vi "Set_Parameter_Instrument (Json).vi"(8 "error in (no error)":errorcluster caption="entrée d'erreur (pas d'erreur)", 10 "Parameter (Json)":string, 11 "Enable_DIO en entrée":refnum<class "Start_Continuous_Ana.lvclass">) -> (0 "error out":errorcluster caption="sortie d'erreur", 3 "Enable_DIO en sortie":refnum<class "Start_Continuous_Ana.lvclass">)   [LabVIEW 2020, in "Library Test.lvlib" / "Start_Continuous_Ana.lvclass"]
uses:
  Start_Continuous_Ana.lvclass
  C:/Users/ngarcin/OneDrive - Altyor/Standard TB/Class/Test/Test (Default)/Test (Default).lvclass
  Ana/Class Ana (Default)/Class Ana (Default).lvclass
  JSON API/JSON Value/Set from JSON string.vi
  JSON API/Variant JSON/Variant to JSON.vi
  JSON API/JSON Value/Get Item by name array.vi
  Test_Wtih_Instr/Test_With_Inst.lvclass
  Instrument/Instrument (Default)/Class Instrument (Default).lvclass
  JSON API/JSON Value/JSON Value.lvclass
  Start_Continuous_Ana.lvclass/Start_Continuous_Ana.ctl
  JSON API/Variant JSON/Variant JSON.lvlib
  JSON API/Get Polymorphic/JSON GetSet.lvlib
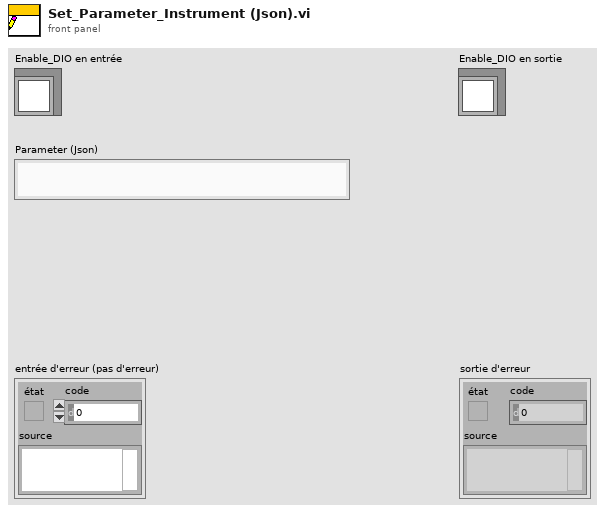
[diagram p1: front panel]
types:
  T1 = cluster{"Device_Com_Port":string, "Rate":u16, "Nb Sample":u16, "Voltage Max":dbl, "Voltage Min":dbl, "Input terminal Configuration":string, "Channel":u8[], "Continuous":bool, "Nb Data_To_Read":i16, "Class Ana":refnum<class "Class Ana (Default).lvclass">}
  T2 = cluster{"Rate":u16, "Nb Sample":u16, "Voltage Max":dbl, "Voltage Min":dbl, "Input terminal Configuration":string, "Channel":u8[], "Nb Data_To_Read":i16}
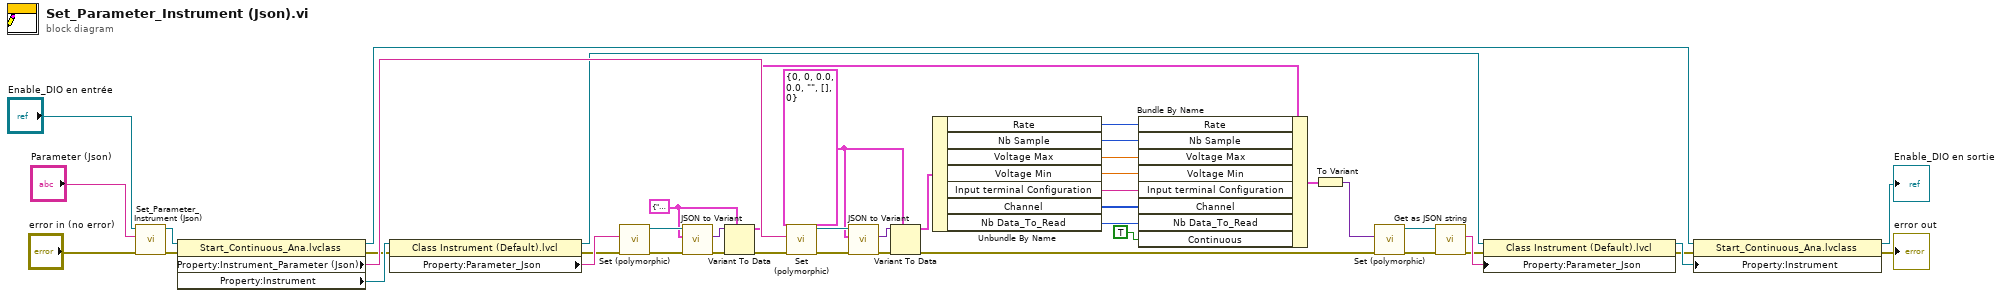
[diagram p0: block diagram]
diagram:
  w6 = T1 {"Device_Com_Port"="", "Rate"=0, "Nb Sample"=0, "Voltage Max"=0.0, "Voltage Min"=0.0, "Input terminal Configuration"="", "Channel"=[], "Continuous"=FALSE, "Nb Data_To_Read"=0, "Class Ana"=refnum} ("Parameter")
  w8 = T2 {"Rate"=0, "Nb Sample"=0, "Voltage Max"=0.0, "Voltage Min"=0.0, "Input terminal Configuration"="", "Channel"=[], "Nb Data_To_Read"=0} ("Parameter")
  n1 = call-parent "Set_Parameter_Instrument (Json).vi"("error in (no error)"="error in (no error)", "Parameter (Json)"="Parameter (Json)", "Test (Default) en entrée"="Enable_DIO en entrée") -> ("error out"=w19:errorcluster, "Test (Default) en sortie"=w27:refnum<class "Start_Continuous_Ana.lvclass">)  [unwired: 7 in]
  n2 = property class="Start_Continuous_Ana.lvclass"(reference=w27, error in=w19) -> (reference out=w23:refnum<class "Start_Continuous_Ana.lvclass">, error out=w18:errorcluster, "Property:Instrument_Parameter (Json)"=w25:string, "Property:Instrument"=w26:refnum<class "Class Instrument (Default).lvclass">)
  n3 = property class="Class Instrument (Default).lvcl"(reference=w26, error in=w18) -> (reference out=w22:refnum<class "Class Instrument (Default).lvclass">, error out=w31:errorcluster, "Property:Parameter_Json"=w33:string)
  n4 = call-poly "Set (polymorphic).vi"("error in (no error)"=w31, "JSON stream"=w33) -> ("error out"=w35:errorcluster, "JSON Value out"=w37:refnum<class "JSON Value.lvclass">)  [unwired: 7 in, 1 out]
  n5 = call "JSON to Variant.vi"("error in (no error)"=w35, "Variant (Data Type)"=w6, "JSON Value"=w37) -> ("error out"=w36:errorcluster, "Variant out"=w34:variant)  [unwired: 7 in]
  n6 = Variant To Data(error in=w36, type=w6, Variant=w34) -> (data=w1:T1, error out=w32:errorcluster)
  n7 = call-poly "Set (polymorphic).vi"("error in (no error)"=w32, "JSON stream"=w25) -> ("error out"=w40:errorcluster, "JSON Value out"=w38:refnum<class "JSON Value.lvclass">)  [unwired: 7 in, 1 out]
  n8 = call "JSON to Variant.vi"("error in (no error)"=w40, "Variant (Data Type)"=w8, "JSON Value"=w38) -> ("error out"=w39:errorcluster, "Variant out"=w41:variant)  [unwired: 7 in]
  n9 = Variant To Data(error in=w39, type=w8, Variant=w41) -> (data=w7:T2, error out=w4:errorcluster)
  n10 = Unbundle By Name(w7) -> ("Rate"=w16:u16, "Nb Sample"=w15:u16, "Voltage Max"=w14:dbl, "Voltage Min"=w13:dbl, "Input terminal Configuration"=w12:string, "Channel"=w11:u8[], "Nb Data_To_Read"=w10:i16)
  n11 = Bundle By Name(cluster=w1, "Rate"=w16, "Nb Sample"=w15, "Voltage Max"=w14, "Voltage Min"=w13, "Input terminal Configuration"=w12, "Channel"=w11, "Nb Data_To_Read"=w10, "Continuous"=TRUE) -> (w5:T1)
  n12 = To Variant(anything=w5) -> (Variant=w29:variant)
  n13 = call-poly "Set (polymorphic).vi"("error in (no error)"=w4, "Variant"=w29) -> ("error out"=w3:errorcluster, "JSON Value out"=w30:refnum<class "JSON Value.lvclass">)  [unwired: 8 in]
  n14 = call "Get as JSON string.vi"("error in (no error)"=w3, "JSON Value in"=w30) -> ("error out"=w2:errorcluster, "<JSON>"=w28:string)  [unwired: 8 in]
  n15 = property class="Class Instrument (Default).lvcl"(reference=w22, error in=w2, "Property:Parameter_Json"=w28) -> (reference out=w24:refnum<class "Class Instrument (Default).lvclass">, error out=w17:errorcluster)
  n16 = property class="Start_Continuous_Ana.lvclass"(reference=w23, error in=w17, "Property:Instrument"=w24) -> (reference out=→"Enable_DIO en sortie":refnum<class "Start_Continuous_Ana.lvclass">, error out=→"error out":errorcluster)
